vi "GetSetBooleanValue.vi"(7 "Set?":bool, 8 "error in (no error)":errorcluster, 9 "Value In":bool, 10 "Name":string, 11 "Camera in":refnum<class "Camera.lvclass">) -> (0 "error out":errorcluster, 1 "Value Out":bool)   [LabVIEW 2020, in "Camera.lvclass"]
uses:
  Camera.lvclass
  Camera.lvclass/Camera.ctl
  bin/gindustrialcam_32-1.dll
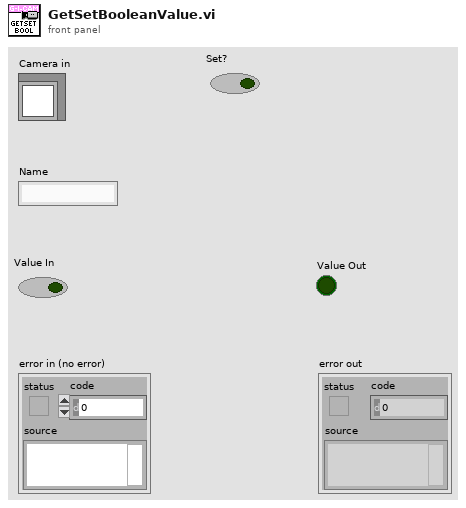
[diagram p1: front panel]
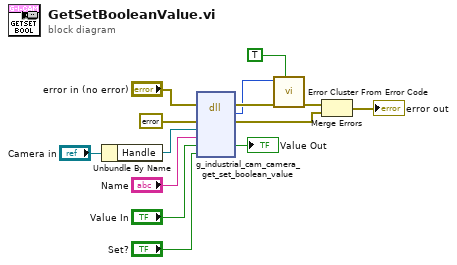
[diagram p0: block diagram]
diagram:
  n1 = Unbundle By Name("Camera in") -> ("Handle"=w3:refnum<data-value>)
  n2 = dll-call lib="C:/Workspace/SSDC/g-industrial-camera/LabVIEW/g_industrial_cam/bin/gindustrialcam_*-1.*" fn="g_industrial_cam_camera_get_set_boolean_value"(error in="error in (no error)", "err"=errorcluster {"status"=FALSE, "code"=0, "source"=""} ("error constant"), "edvr"=w3, "name"="Name", "value"="Value In", "set"="Set?") -> (error out=w14:errorcluster, "Mg_Error"=w13:i32, "err"=w11:errorcluster, "value"=→"Value Out":bool)  [unwired: 5 in, 1 out]
  n3 = call <vilib>:"Error Cluster From Error Code.vi"("show call chain? (False)"=TRUE, "error in (no error)"=w14, "error code (0)"=w13) -> ("error out"=w12:errorcluster)  [unwired: 6 in]
  n4 = Merge Errors(w12, w11) -> (→"error out":errorcluster)
